vi "Move to next focus state.vi"(8 "error in":errorcluster, 10 "Next state indicator":string, 11 "VISA resource in":refnum<visa-resource-name>) -> (0 "error out":errorcluster, 1 "LED TOO DIM?":bool, 3 "VISA resource out":refnum<visa-resource-name>)   [LabVIEW 2018]
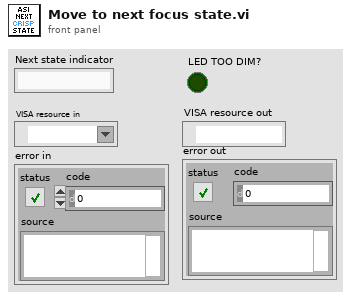
[diagram p1: front panel]
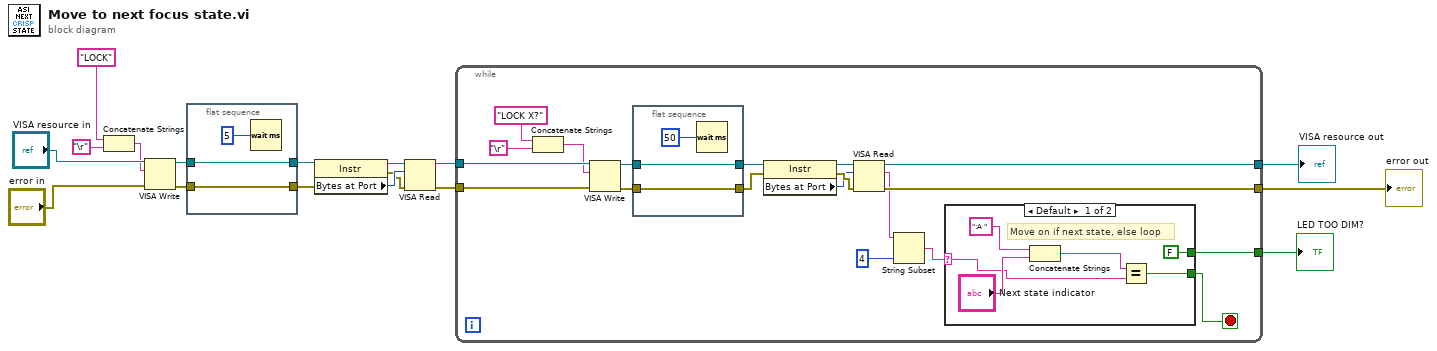
[diagram p0: block diagram]
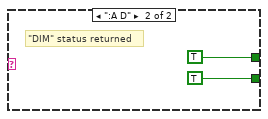
[diagram p2: hidden frame]
diagram:
  n1 = Concatenate Strings("LOCK" ("write buffer"), "\r") -> (w2:string)
  n2 = VISA Write(VISA resource name="VISA resource in", write buffer=w2, error in (no error)="error in") -> (VISA resource name out=w12:refnum<visa-resource-name>, error out=w13:errorcluster)  [unwired: 1 out]
  n3 = flat-sequence {
    tunnel: [w20] -> w15
    tunnel: w12 -> [w20]
    tunnel: [w18] -> w14
    tunnel: w13 -> [w18]
    frame #0 {
      n4 = Wait (ms)(milliseconds to wait=u32 5) -> ()  [unwired: 1 out]
    }
  }
  n5 = property class="Instr"(reference=w15, error in=w14) -> (reference out=w11:refnum<visa-resource-name>, error out=w9:errorcluster, "Bytes at Port"=w10:u32)
  n6 = VISA Read(VISA resource name=w11, byte count=w10, error in (no error)=w9) -> (VISA resource name out=w16:refnum<visa-resource-name>, error out=w17:errorcluster)  [unwired: 2 out]
  n7 = while {
    tunnel: w16 -> [w39]
    tunnel: w17 -> [w38]
    tunnel: [w30] -> w5
    tunnel: [w29] -> w6
    tunnel: [w21] -> w1
    stop <- w22 stop-if-true
    n8 = Concatenate Strings("LOCK X?" ("write buffer"), "\r") -> (w26:string)
    n9 = VISA Write(VISA resource name=w39, write buffer=w26, error in (no error)=w38) -> (VISA resource name out=w36:refnum<visa-resource-name>, error out=w37:errorcluster)  [unwired: 1 out]
    n10 = flat-sequence {
      tunnel: [w50] -> w31
      tunnel: w36 -> [w50]
      tunnel: [w48] -> w32
      tunnel: w37 -> [w48]
      frame #0 {
        n11 = Wait (ms)(milliseconds to wait=u32 50) -> ()  [unwired: 1 out]
      }
    }
    n12 = property class="Instr"(reference=w31, error in=w32) -> (reference out=w33:refnum<visa-resource-name>, error out=w35:errorcluster, "Bytes at Port"=w34:u32)
    n13 = VISA Read(VISA resource name=w33, byte count=w34, error in (no error)=w35) -> (VISA resource name out=w30:refnum<visa-resource-name>, read buffer=w24:string, error out=w29:errorcluster)  [unwired: 1 out]
    n14 = String Subset(string=w24, length (rest)=4 ("length (rest)")) -> (substring=w23:string)  [unwired: 1 in]
    n15 = case shown="Default" w23 {
      selector: w23 -> [w42 _]
      tunnel: [w41 TRUE] -> w22
      tunnel: [FALSE TRUE] -> w21
      frame Default {
        # "Move on if next state, else loop"
        n16 = Concatenate Strings(":A " ("string"), "Next state indicator") -> (w43:string)
        n17 = Equal?(x=w43, y=w42) -> (x = y?=w41:bool)
      }
      frame ":A D" {
        # "\"DIM\" status returned"
      }
    }
  }
  "error out" <- w6
  "VISA resource out" <- w5
  "LED TOO DIM?" <- w1
